vi "Add Device.vi"(8 "error in (no error)":errorcluster, 10 "Device":refnum<class "Device.lvclass">, 11 "DeviceListPanel in":refnum<class "DeviceListPanel.lvclass">) -> (0 "error out":errorcluster, 3 "DeviceListPanel out":refnum<class "DeviceListPanel.lvclass">)   [LabVIEW 2020, in "PicoG-App.lvlib" / "DeviceListPanel.lvclass"]
uses:
  DeviceListPanel.lvclass
  Device/Device.lvclass
  DeviceListPanel.lvclass/DeviceListPanel.ctl
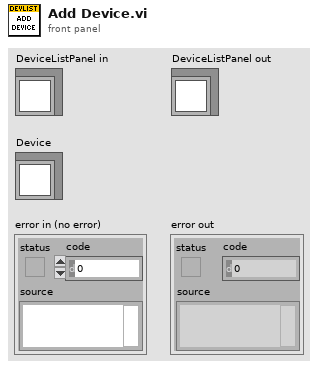
[diagram p1: front panel]
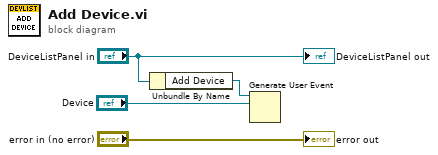
[diagram p0: block diagram]
diagram:
  n1 = Unbundle By Name("DeviceListPanel in") -> ("Add Device"=w2:refnum<user-event>)
  n2 = Generate User Event(user event=w2, event data cluster="Device") -> ()  [unwired: 2 in, 2 out]
  "error out" <- "error in (no error)"
  "DeviceListPanel out" <- "DeviceListPanel in"
